vi "NXT Create tug array C.vi"(2 "Local Heading":i16 step=10) -> (0 "FB array":i16[](array[numeric]))   [LabVIEW 2012]
doc: "This VI accepts the present boat Heading and the desired boat Heading to the new way point and a 16 bit integer as the desired velocity. It returns a 16 bit array 16 long which is used by the MidBrain Arbiter. In doing so a shift is made from global to local corridinate system. The output array represents angles in the local corridinate system."
uses:
  <vilib>/NXT/Dual Mode Library/prims/inRangeAndCoerce/inRangeAndCoerce_int.vi
panel:
  out "FB array":cluster{i32, i32, i16[]}(graph)
  out "Right?":bool
  out "Heading\nIndex":i16
  # "15"
  # "0"
  # "7"
  # "8"
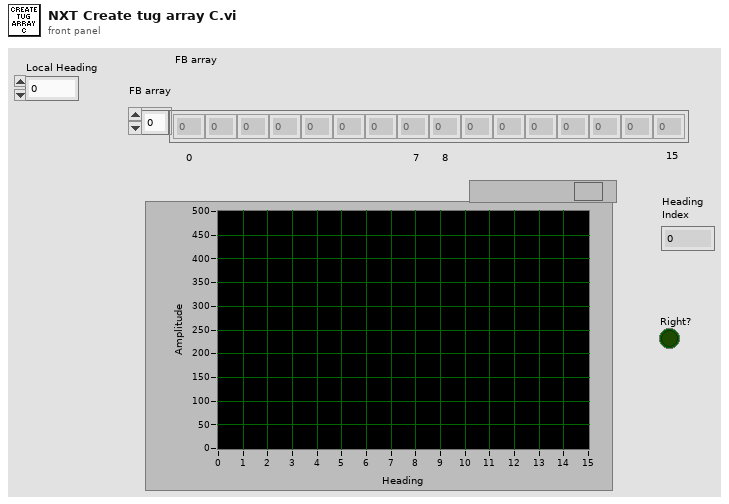
[diagram p1: front panel]
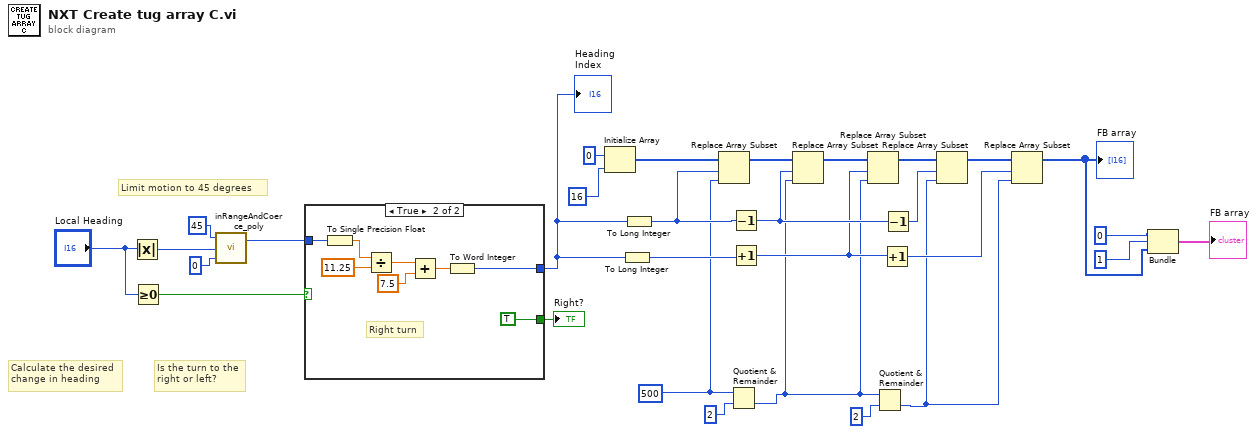
[diagram p0: block diagram]
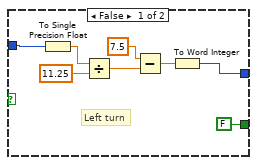
[diagram p2: hidden frame]
diagram:
  w4 = i16 500 ("y")
  # "Limit motion to 45 degrees"
  # "Is the turn to the\nright or left?"
  # "Calculate the desired\nchange in heading"
  n1 = Absolute Value(x="Local Heading") -> (abs(x)=w3:i16)
  n2 = Greater Or Equal To 0?(x="Local Heading") -> (x >= 0?=w1:bool)
  n3 = call-poly <vilib>:"inRangeAndCoerce_poly.vi"("lower limit"=0, "x"=w3, "upper limit"=45) -> ("coerced(x)"=w13:i32)  [unwired: 1 out]
  n4 = case shown="True" w1 {
    tunnel: w13 -> [w35 w46]
    tunnel: [w32 w40] -> w11
    tunnel: [FALSE TRUE] -> w9
    frame False {
      # "Left turn"
      n5 = To Single Precision Float(number=w35) -> (single precision float=w36:sgl)
      n6 = Divide(x=w36, y=sgl 11.25) -> (x/y=w34:sgl)
      n7 = Subtract(x=sgl 7.5 ("y"), y=w34) -> (x-y=w38:sgl)
      n8 = To Word Integer(number=w38) -> (16bit integer=w32:i16)
    }
    frame True {
      # "Right turn"
      n9 = To Single Precision Float(number=w46) -> (single precision float=w45:sgl)
      n10 = Divide(x=w45, y=sgl 11.25) -> (x/y=w43:sgl)
      n11 = Add(x=w43, y=sgl 7.5) -> (x+y=w41:sgl)
      n12 = To Word Integer(number=w41) -> (16bit integer=w40:i16)
    }
  }
  "Heading\nIndex" <- w11
  "Right?" <- w9
  n13 = Initialize Array(i16 0 ("element"), 16 ("dimension size")) -> (w28:i16[])
  n14 = To Long Integer(number=w11) -> (32bit integer=w12:i32)
  n15 = To Long Integer(number=w11) -> (32bit integer=w10:i32)
  n16 = Replace Array Subset(array=w28, new element=w4, index=w10) -> (w27:i16[])
  n17 = Quotient & Remainder(x=w4, y=i16 2) -> (floor(x/y)=w17:i16)  [unwired: 1 out]
  n18 = Decrement(x=w10) -> (x-1=w22:i32)
  n19 = Increment(x=w12) -> (x+1=w20:i32)
  n20 = Replace Array Subset(array=w27, new element=w17, index=w22) -> (w26:i16[])
  n21 = Replace Array Subset(array=w26, new element=w17, index=w20) -> (w23:i16[])
  n22 = Quotient & Remainder(x=w17, y=i16 2) -> (floor(x/y)=w16:i16)  [unwired: 1 out]
  n23 = Increment(x=w20) -> (x+1=w19:i32)
  n24 = Decrement(x=w22) -> (x-1=w21:i32)
  n25 = Replace Array Subset(array=w23, new element=w16, index=w21) -> (w24:i16[])
  n26 = Replace Array Subset(array=w24, new element=w16, index=w19) -> (w6:i16[])
  "FB array" <- w6
  n27 = Bundle(0, 1, w6) -> (→"FB array":cluster{i32, i32, i16[]})  [unwired: 1 in]
